vi "C8855-01_NumForming.vi"(10 "In":u32) -> (3 "Out":string)   [LabVIEW 2017]
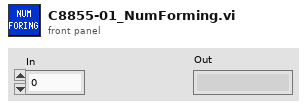
[diagram p1: front panel]
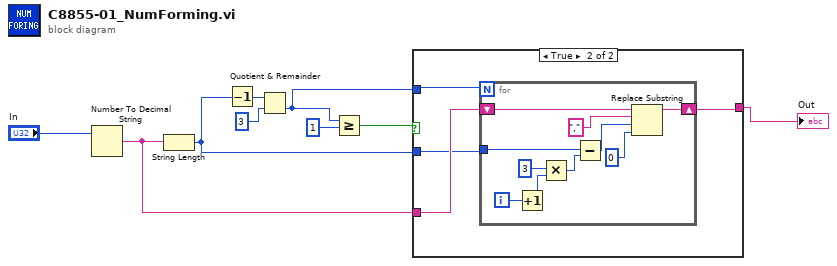
[diagram p0: block diagram]
diagram:
  n1 = Number To Decimal String(number="In") -> (decimal integer string=w5:string)  [unwired: 1 in]
  n2 = String Length(string=w5) -> (length=w1:i32)
  n3 = Decrement(x=w1) -> (x-1=w2:i32)
  n4 = Quotient & Remainder(x=w2, y=3) -> (floor(x/y)=w6:i32)  [unwired: 1 out]
  n5 = Greater Or Equal?(x=w6, y=1) -> (x >= y?=w3:bool)
  n6 = case shown="True" w3 {
    tunnel: w6 -> [_ w11]
    tunnel: w5 -> [w10 w14]
    tunnel: [w10 w12] -> w4
    tunnel: w1 -> [_ w13]
    frame False {
    }
    frame True {
      n7 = for {
        N: w11 -> [_]
        tunnel: w13 -> [w19]
        shift-right: [w15] -> w12
        shift-left: w14 -> [w24]
        i -> [w21]
        n8 = Increment(x=w21) -> (x+1=w20:i32)
        n9 = Multiply(x=3, y=w20) -> (x*y=w18:i32)
        n10 = Subtract(x=w19, y=w18) -> (x-y=w17:i32)
        n11 = Replace Substring(2:0, 3:w17, 4:",", 5:w24) -> (1:w15:string)  [unwired: 1 out]
      }
    }
  }
  "Out" <- w4
